vi "Single_IMU_gaitR.vi"() -> ()   [LabVIEW 2022 SP3]
uses:
  <vilib>/Platform/TimedLoop/XDataNode/wakeup.ctl
  <vilib>/Platform/TimedLoop/XDataNode/XDNodeRunTimeDep.lvlib
  <vilib>/Platform/TimedLoop/XDataNode/nitl_modes.ctl
  <vilib>/Platform/TimedLoop/XDataNode/timing_clust.ctl
  <vilib>/Platform/TimedLoop/XDataNode/XDataNode.xnode
  <vilib>/Analysis/NI_AALBase.lvlib
  <vilib>/Analysis/Matrix/Datatypes/RealMatrix.ctl
  <vilib>/Analysis/Matrix/NI_Matrix.lvlib
panel:
  in  "STOP":bool
  out "FootACC":sgl[](array[numeric])
  out "Foot Real Matrix":T1
  out "Step":cluster{i32}(graph)
  out "Corrected ACC":dbl[](array[numeric])
  in  "?":bool
  # "Tips:"
  # "SWING Phase --> 1\nSTANCE Phase -->0\nBased on SINGLE IMU Plased on the Foot"
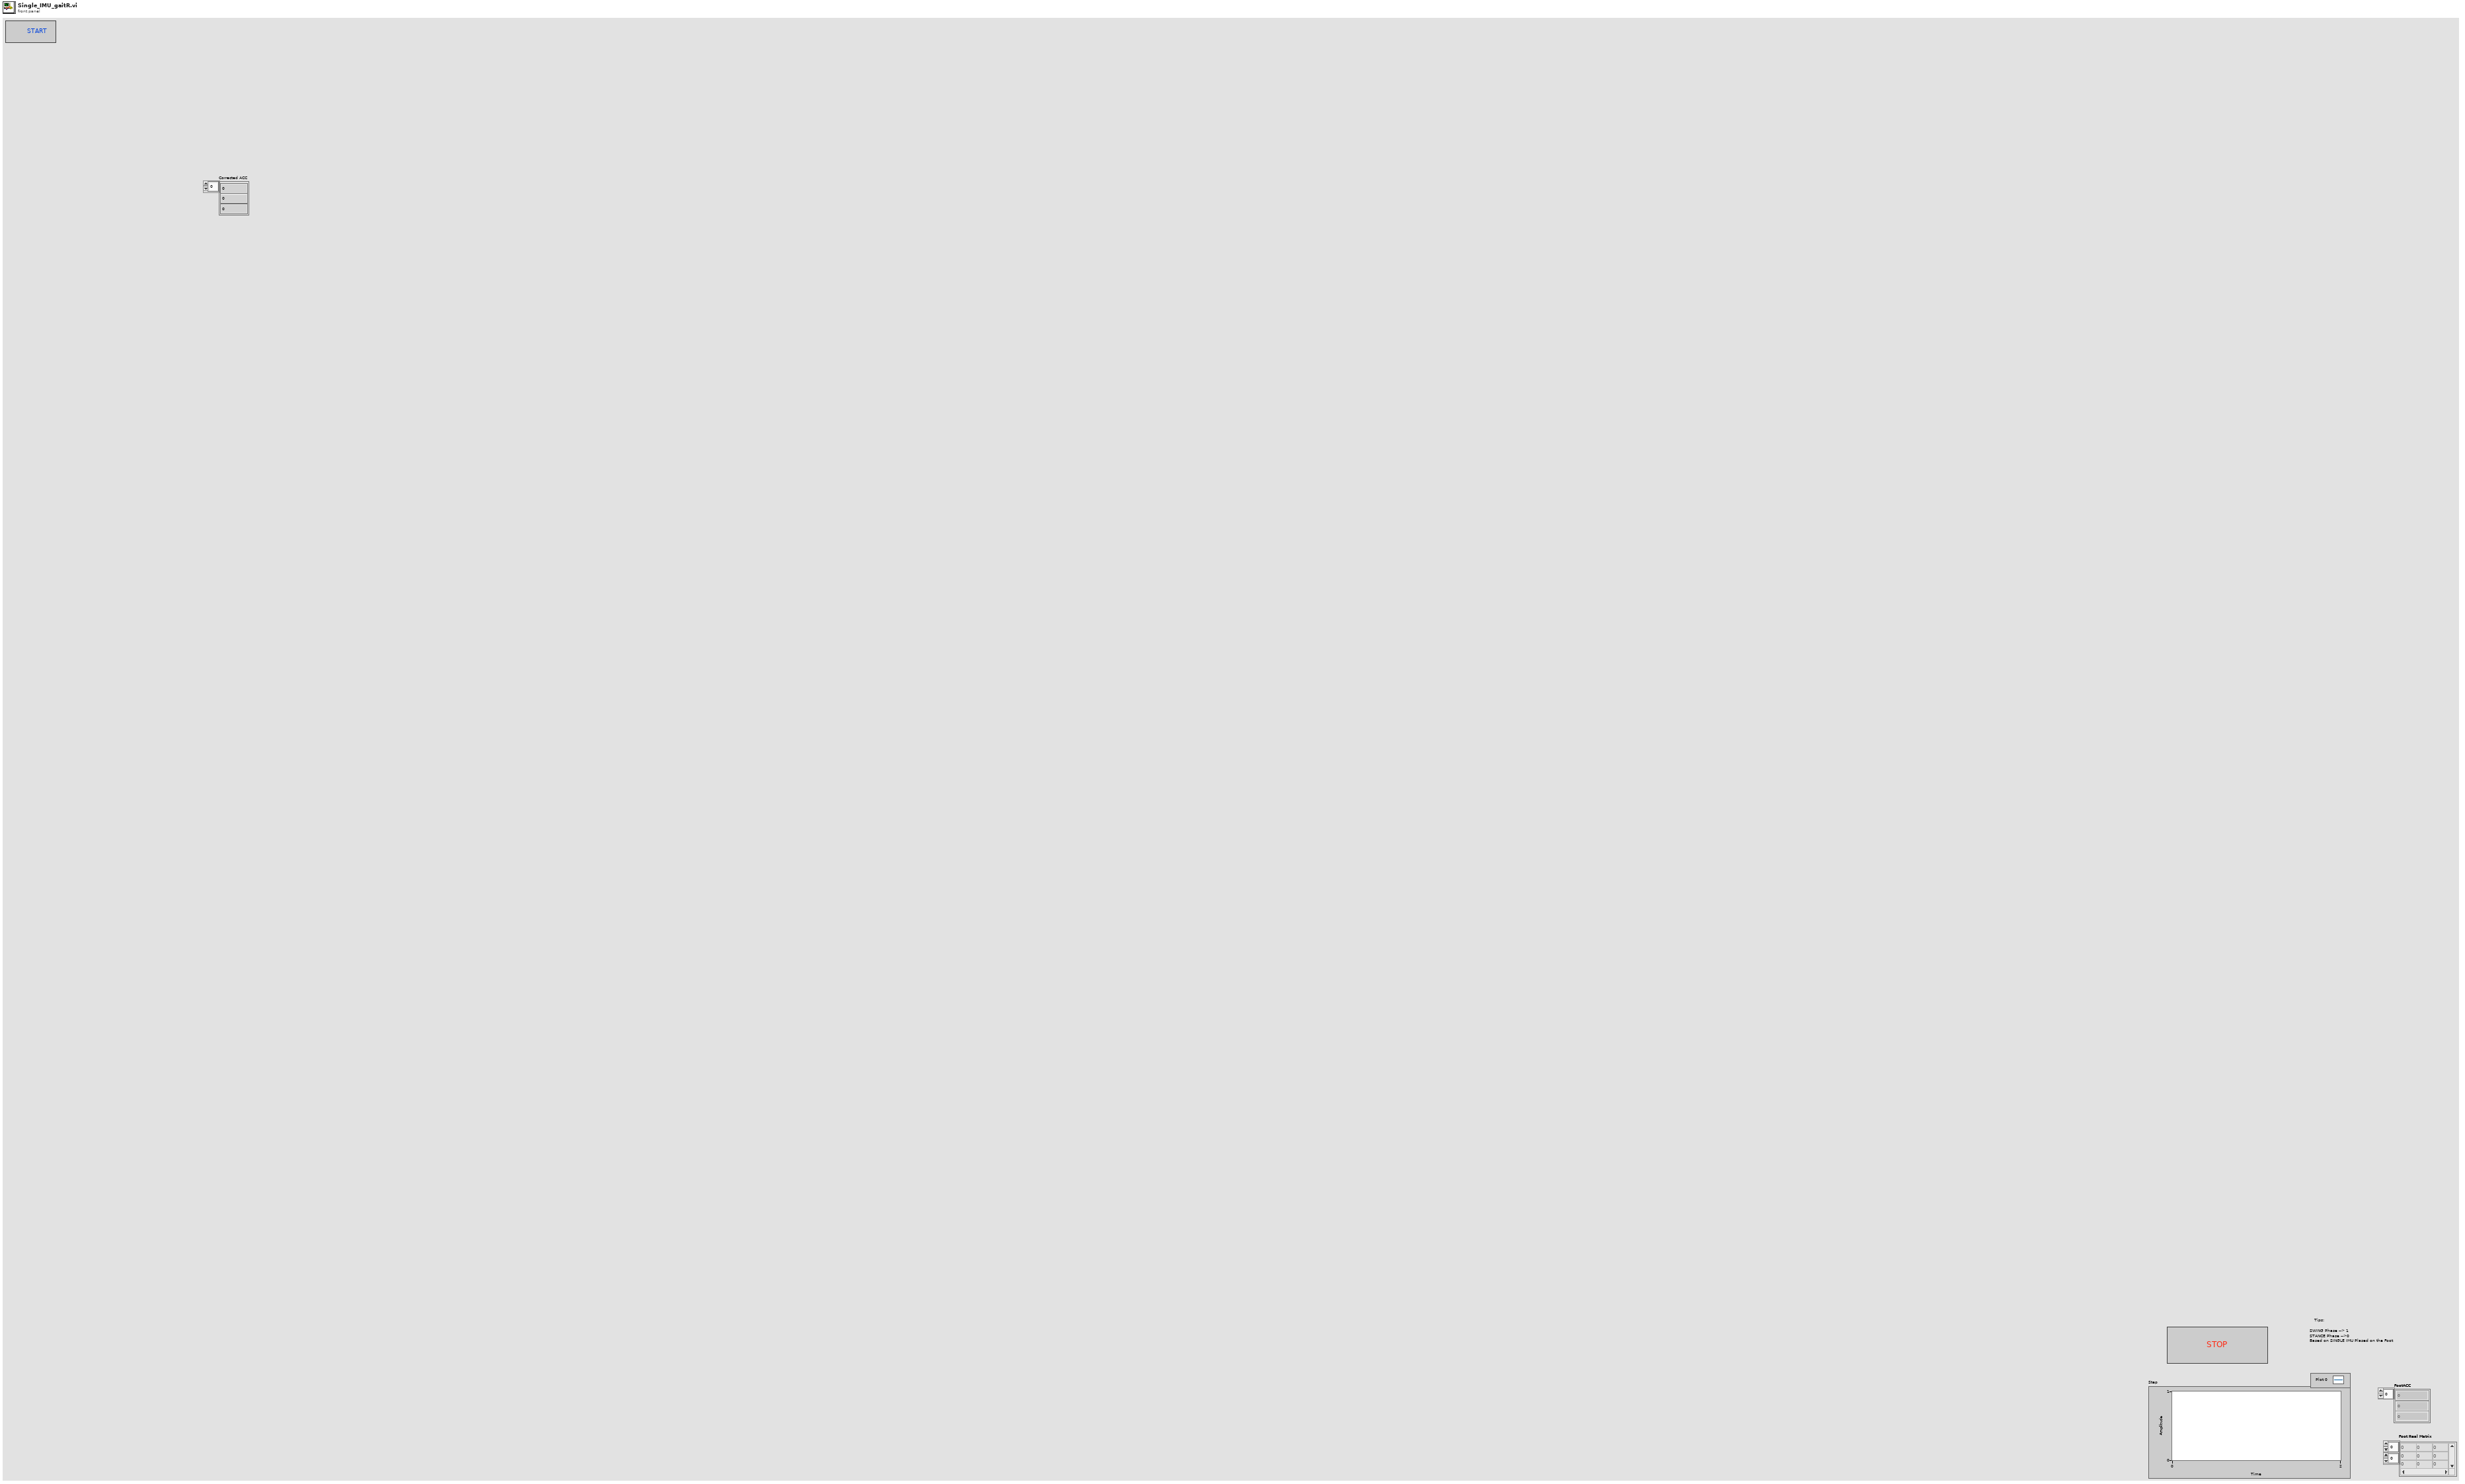
[diagram p1: front panel]
types:
  T1 = typedef "NI_Matrix.lvlib/RealMatrix.ctl" = dbl[][]
  T2 = typedef "XDNodeRunTimeDep.lvlib/timing_clust.ctl" = cluster{"Expected End [f-1]":u64, "Actual End [f-1]":u64, "Finished Late? [f-1]":bool, "Expected End [i-1]":u64, "Actual End [i-1]":u64, "Finished Late? [i-1]":bool, "Expected Start [i]":u64, "Actual Start [i]":u64, "Expected Start [f]":u64, "Actual Start [f]":u64, "Source Name":string, "Structure Name":string, "Period":i64, "Deadline":i64, "Offset":i64, "Start":i64, "Priority":i32, "Timeout":i32, "Mode":T3, "Wakeup Reason":T4, "Error":errorcluster, "Source Type":string, "Secondary Source Type":string, "Global End Time":u64, "Global Start Time":u64, "Frame Duration":u64, "Iteration Duration":u64, "Assigned CPU":i32, "I/O Scan Engine Mode":u32}
  T3 = typedef "XDNodeRunTimeDep.lvlib/nitl_modes.ctl" = enum32{"No Change", "Process missed periods, maintain original phase", "Discard missed periods, maintain original phase", "Process missed periods, ignore original phase", "Discard missed periods, ignore original phase"}
  T4 = typedef "XDNodeRunTimeDep.lvlib/wakeup.ctl" = enum32{"Normal", "Aborted", "Asynchronous wakeup", "Timing source error", "Timed loop error", "Timeout"}
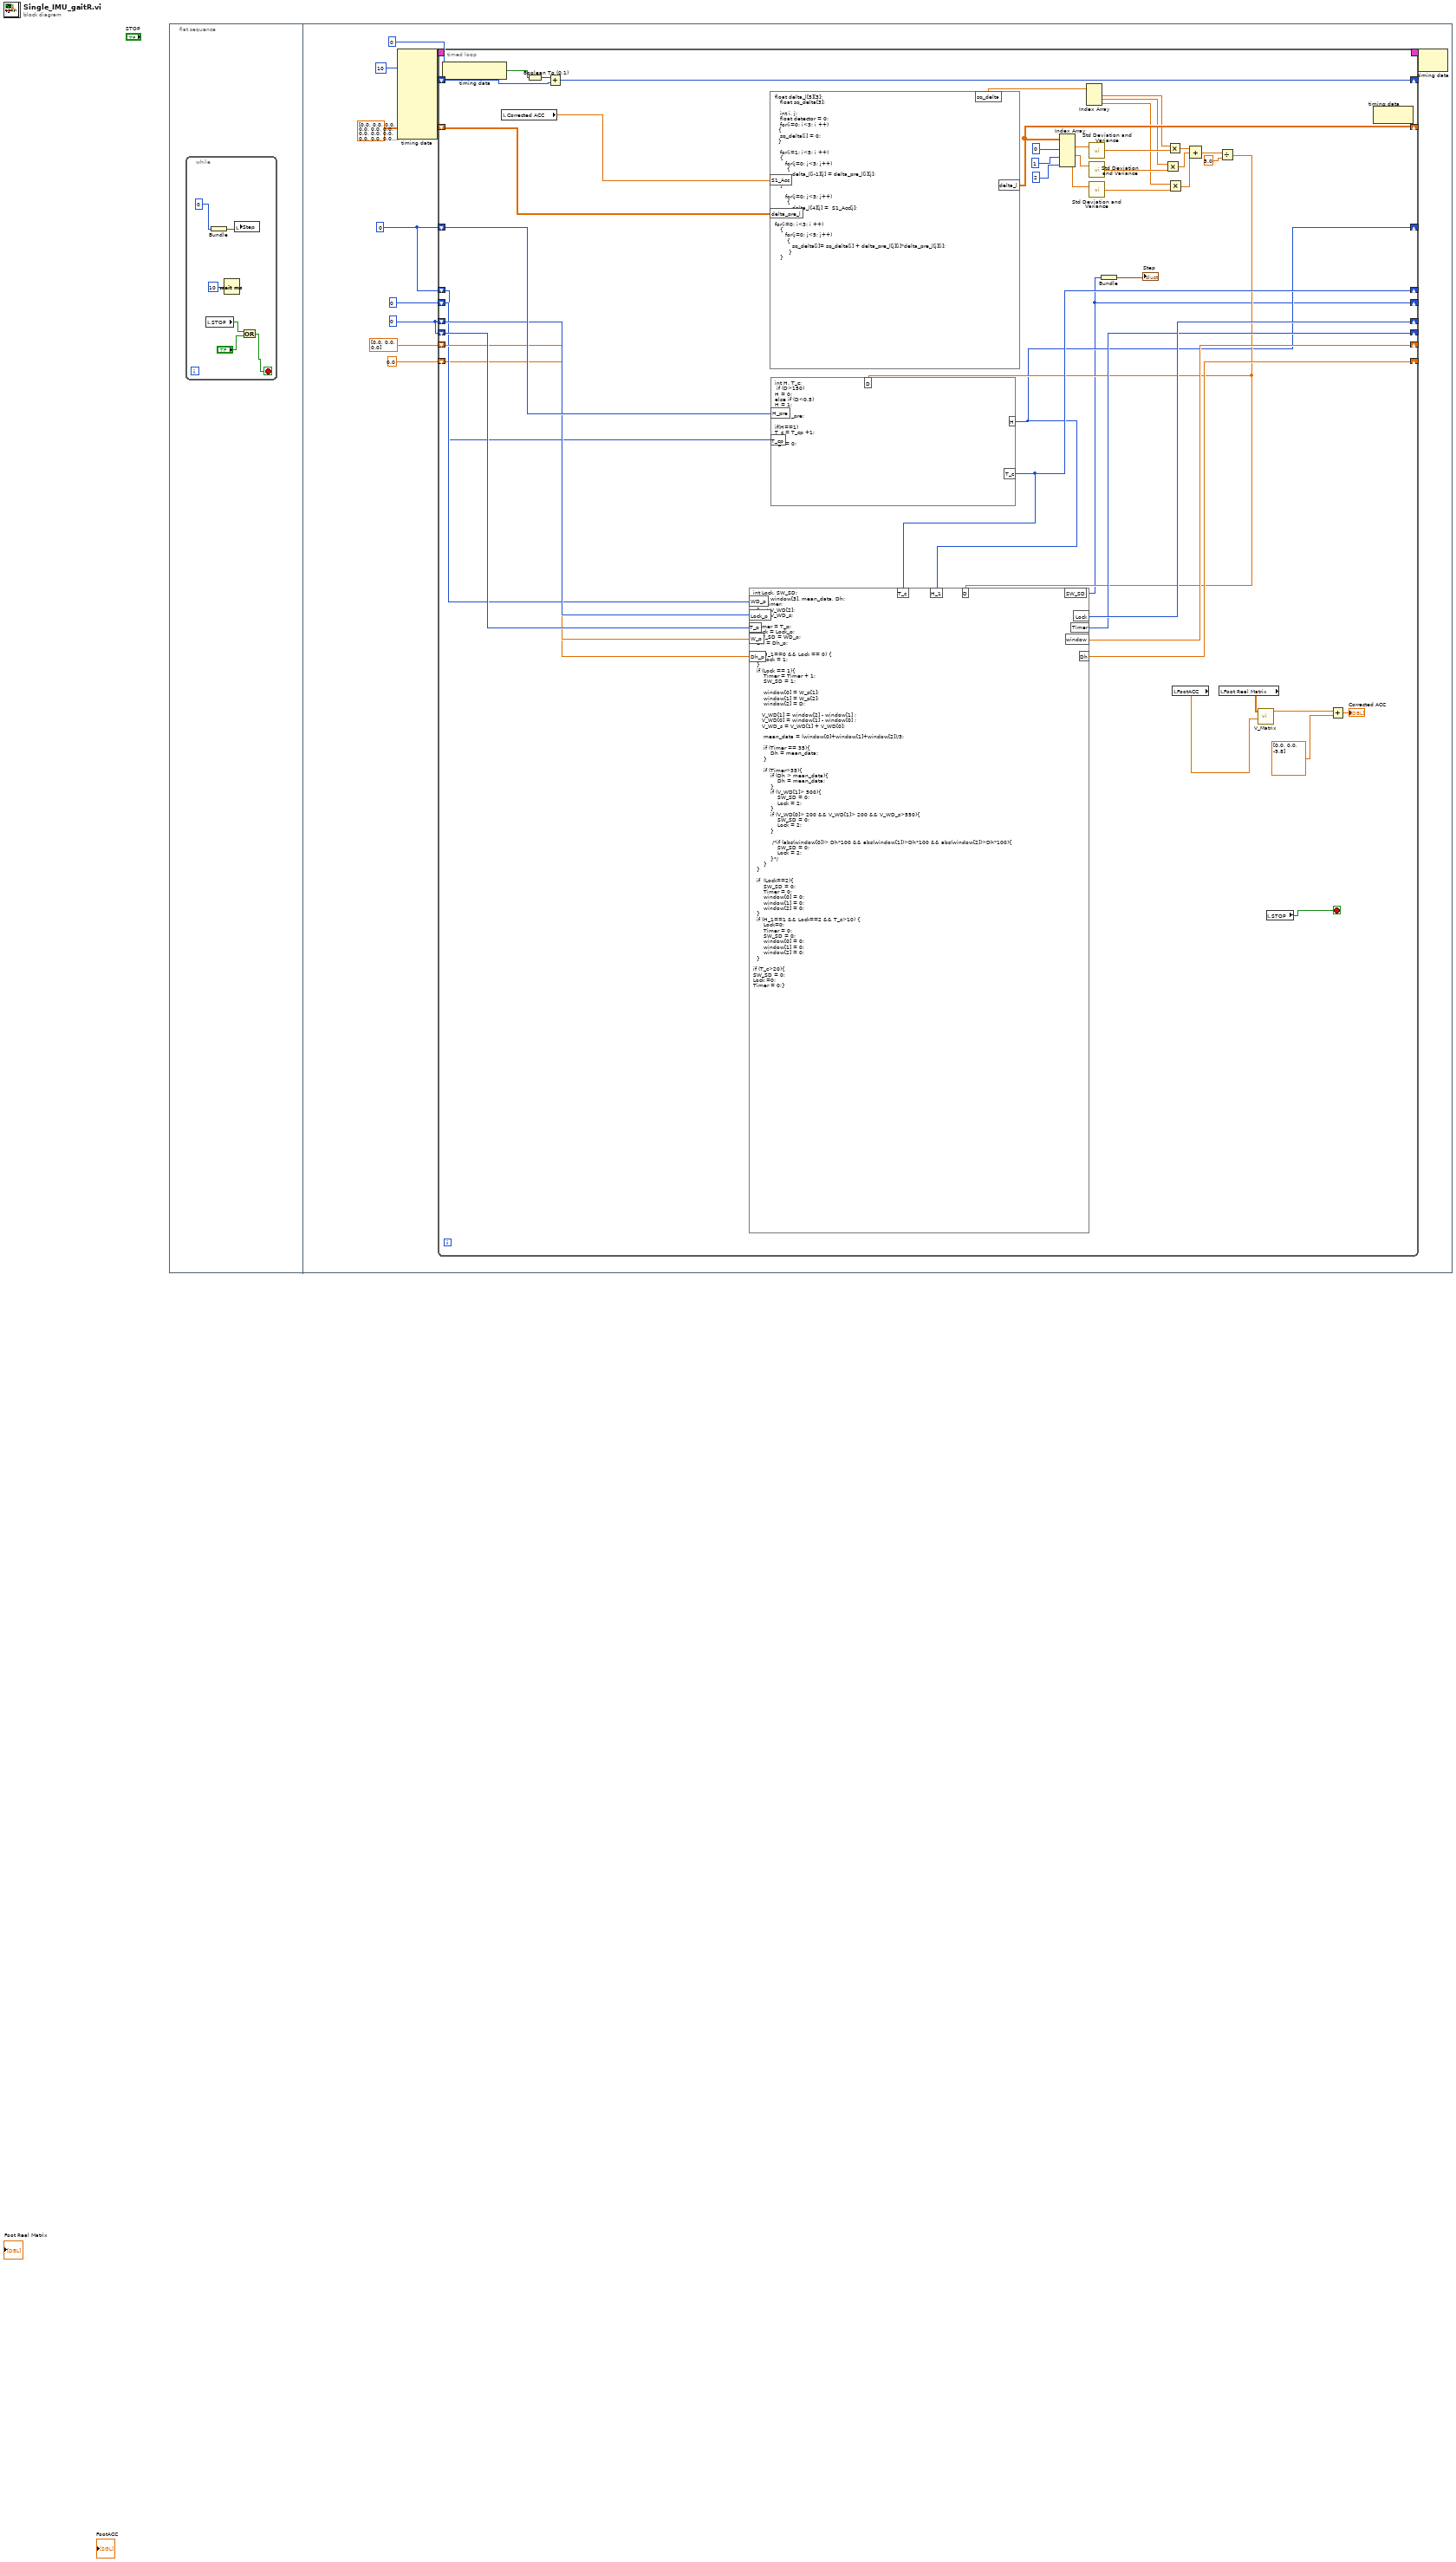
[diagram p0: block diagram]
diagram:
  n1 = flat-sequence {
    frame #0 {
      n2 = while {
        stop <- w4 stop-if-true
        n3 = local read "STOP"() -> (w3:bool)
        n4 = Bundle("milliseconds to wait"=u32 0) -> (w2:cluster{"milliseconds to wait":u32})  [unwired: 1 in]
        n5 = Wait (ms)(milliseconds to wait=u32 10) -> ()  [unwired: 1 out]
        n6 = local write "Step"(w2) -> ()
        n7 = Or(x=w3, y="?") -> (x .or. y?=w4:bool)
      }
    }
    frame #1 {
      w10 = 0
      w8 = 0
      n8 = node-c288(i64 10 ("Period")) -> (w16:T2)  [unwired: 9 in]
      n9 = timed-loop {
        timing: w16 -> [_]
        timing-out: [_] -> w15
        shift-right: [w57] -> _
        shift-left: dbl[][] [[0.0, 0.0, 0.0], [0.0, 0.0, 0.0], [0.0, 0.0, 0.0], [0.0, 0.0, 0.0], [0.0, 0.0, 0.0], [0.0, 0.0, 0.0], [0.0, 0.0, 0.0], [0.0, 0.0, 0.0]] -> [w63]
        shift-right: [w60] -> _
        shift-left: i16 0 -> [w59]
        shift-right: [w18] -> _
        shift-left: w8 -> [w45]
        shift-right: [w44] -> _
        shift-left: w10 -> [w43]
        shift-right: [w42] -> _
        shift-left: w10 -> [w41]
        shift-right: [w40] -> _
        shift-left: dbl[] [0.0, 0.0, 0.0] -> [w39]
        shift-right: [w17] -> _
        shift-left: 0 -> [w38]
        shift-right: [w29] -> _
        shift-left: w8 -> [w21]
        shift-right: [w28] -> _
        shift-left: 0.0 -> [w27]
        stop <- w58 stop-if-true
        n10 = node-c288() -> (w62:bool)  [unwired: 1 in]
        n11 = local read "Corrected ACC"() -> (w20:dbl[])
        n12 = Boolean To (0,1)(Boolean=w62) -> (0, 1=w61:i16)
        n13 = Add(x=w61, y=w59) -> (x+y=w60:i16)
        n14 = formula code="float delta_l[5][3];\n   float sq_delta[3];\n\n   int i, j; \n   float detector = 0;\n   for(i=0; i<3; i ++)\n  {\n   sq_delta[i] = 0;\n  }\n\n   for(i=1; i<5; i ++)\n   {\n      for(j=0; j<3; j++)\n       { \n          delta_l[i-1][j] = delta_pre_l[i][j];\n        }\n   }\n\n      for(j=0; j<3; j++)\n       { \n          delta_l[4][j] =  S1_Acc[j];\n        }\n\nfor(i=0; i<3; i ++)\n   {\n      for(j=0; j<5; j++)\n       { \n          sq_delta[i]= sq_delta[i] + delta_pre_l[j][i]*delta_pre_l[j][i];\n        }\n   }"("S1_Acc"=w20, "delta_pre_l"=w63) -> ("delta_l"=w57:dbl[][], "sq_delta"=w34:dbl[])
        n15 = Index Array(array=w57, index (col) #1=0 ("disabled index (col)"), index (col) #2=1 ("index (col)"), index (col) #3=2 ("index (col)")) -> (element #1=w55:dbl[], element #2=w52:dbl[], element #3=w51:dbl[])  [unwired: 3 in]
        n16 = Index Array(array=w34) -> (element #1=w33:dbl, element #2=w32:dbl, element #3=w31:dbl)  [unwired: 3 in]
        n17 = call <vilib>:"Std Deviation and Variance.vi"("X"=w55) -> ("standard deviation"=w35:dbl)  [unwired: 1 in, 2 out]
        n18 = call <vilib>:"Std Deviation and Variance.vi"("X"=w52) -> ("standard deviation"=w50:dbl)  [unwired: 1 in, 2 out]
        n19 = call <vilib>:"Std Deviation and Variance.vi"("X"=w51) -> ("standard deviation"=w49:dbl)  [unwired: 1 in, 2 out]
        n20 = Multiply(x=w32, y=w50) -> (x*y=w47:dbl)
        n21 = Multiply(x=w33, y=w35) -> (x*y=w48:dbl)
        n22 = Multiply(x=w31, y=w49) -> (x*y=w46:dbl)
        n23 = local read "FootACC"() -> (w25:sgl[])
        n24 = Compound Arithmetic op=ADD(w48, w47, w46) -> (w37:dbl)
        n25 = local read "Foot Real Matrix"() -> (w26:T1)
        n26 = Divide(x=w37, y=5.0) -> (x/y=w19:dbl)
        n27 = formula code="int H, T_c;\n if (D>150)\nH = 0;\nelse if (D<0.5)\nH = 1;\nelse \nH = H_pre;\n\nif(H==1)\nT_c = T_cp +1;\nelse\nT_c = 0;"("D"=w19, "H_pre"=w45, "T_cp"=w21) -> ("H"=w18:i32, "T_c"=w29:i32)
        n28 = formula code="int Lock, SW_SD;\n  float window[3], mean_data, Dh;\n  int Timer;\n  float V_WD[2];\n  float V_WD_s;\n\n  Timer = T_p;\n  Lock = Lock_p;\n  SW_SD = WD_p;\n  Dh = Dh_p;\n\n  if (H_1==0 && Lock == 0) {\n      Lock = 1;\n  }\n  if (Lock == 1){\n      Timer = Timer + 1;\n      SW_SD = 1;\n      \n      window[0] = W_p[1];\n      window[1] = W_p[2];\n      window[2] = D;\n      \n     V_WD[1] = window[2] - window[1] ;\n     V_WD[0] = window[1] - window[0] ;\n     V_WD_s = V_WD[1] + V_WD[0];\n\n      mean_data = (window[0]+window[1]+window[2])/3;\n\n      if (Timer == 35){\n          Dh = mean_data;\n      }\n\n      if (Timer>35){\n          if (Dh > mean_data){\n              Dh = mean_data;\n          }\n          if (V_WD[1]> 500){\n              SW_SD = 0;\n              Lock = 2;\n          }\n          if (V_WD[0]> 200 && V_WD[1]> 200 && V_WD_s>550){\n              SW_SD = 0;\n              Lock = 2;\n          }\n        \n           /*if (abs(window[0])> Dh*100 && abs(window[1])>Dh*100 && abs(window[2])>Dh*100){\n              SW_SD = 0;\n              Lock = 2;\n          }*/\n      }\n  }\n  \n  if  (Lock==2){ \n      SW_SD = 0;\n      Timer = 0;\n      window[0] = 0;\n      window[1] = 0;\n      window[2] = 0;\n  }\n  if (H_1==1 && Lock==2 && T_c>10) {\n      Lock=0;\n      Timer = 0;\n      SW_SD = 0;\n      window[0] = 0;\n      window[1] = 0;\n      window[2] = 0;\n  }\n\nif (T_c>20){\nSW_SD = 0;\nLock =0;\nTimer = 0;}"("D"=w19, "H_1"=w18, "Lock_p"=w43, "T_p"=w41, "W_p"=w39, "WD_p"=w38, "T_c"=w29, "Dh_p"=w27) -> ("SW_SD"=w17:i32, "Lock"=w44:i32, "Timer"=w42:i32, "window"=w40:dbl[], "Dh"=w28:dbl)
        n29 = Bundle(w17) -> (→"Step":cluster{i32})  [unwired: 1 in]
        n30 = call "V_Matrix.vi"("V"=w25, "M"=w26) -> ("V_o"=w22:dbl[])  [unwired: 9 in]
        n31 = local read "STOP"() -> (w58:bool)
        n32 = Add(x=w22, y=dbl[] [0.0, 0.0, -9.8] ("V")) -> (x+y=→"Corrected ACC":dbl[])
        n33 = node-c288() -> ()  [unwired: 1 in, 1 out]
      }
      n34 = node-c288(w15) -> ()  [unwired: 1 out]
    }
  }
